vi "ClearResults.vi"   [LabVIEW 2011]
uses:
  qtrk/QTrkLVBinding/ResultManagerInstance.ctl
  GlobalVariables.vi
types:
  T1 = typedef "ResultManagerInstance.ctl" = cluster{"InstancePtr":u64}
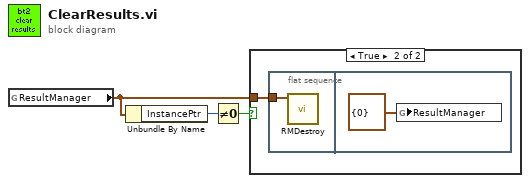
[diagram p0: block diagram]
diagram:
  n1 = global read "GlobalVariables.vi" "ResultManager"() -> (w1:T1)
  n2 = Unbundle By Name(w1) -> ("InstancePtr"=w2:u64)
  n3 = Not Equal To 0?(x=w2) -> (x != 0?=w3:bool)
  n4 = case shown="True" w3 {
    tunnel: w1 -> [_ w4]
    frame False {
    }
    frame True {
      n5 = flat-sequence {
        tunnel: w4 -> [w5]
        frame #0 {
          n6 = call "RMDestroy.vi"("ResultManager"=w5) -> ()  [unwired: 9 in, 2 out]
        }
        frame #1 {
          n7 = global write "GlobalVariables.vi" "ResultManager"(T1 {"InstancePtr"=0} ("ResultManager")) -> ()
        }
      }
    }
  }
